vi "TCP Send Recieve.vi"(6 "bytes to read":i32=-1, 7 "mode (standard)":T1(ring), 8 "Error In":errorcluster, 9 "timeout ms (25000)":i32=25000, 10 "data in":string, 11 "connection ID":refnum<k5>) -> (0 "Error Out":errorcluster, 1 "bytes written":i32, 2 "data out":string, 3 "connection ID out":refnum<k5>)   [LabVIEW 2024]
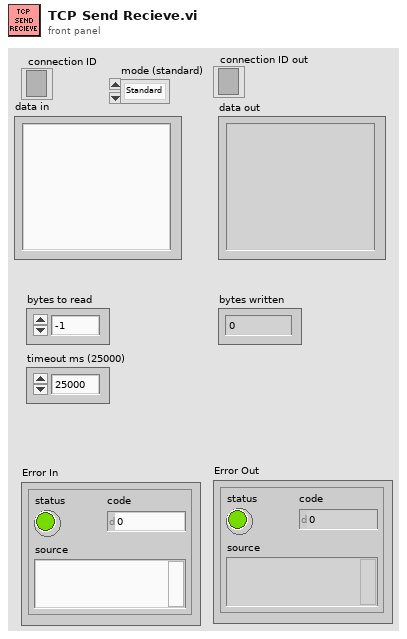
[diagram p1: front panel]
types:
  T1 = enum16{"Standard", "Buffered", "CRLF", "Immediate"}
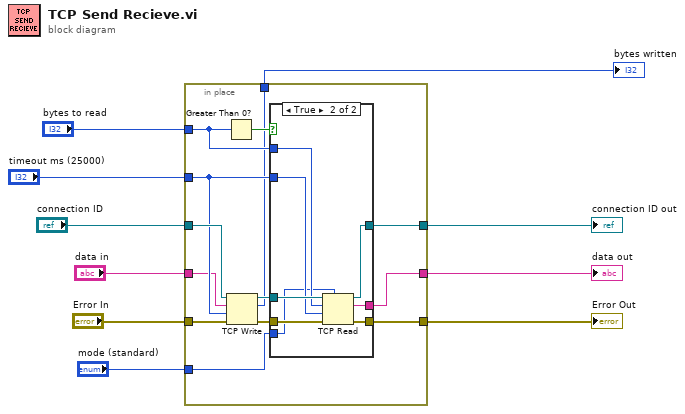
[diagram p0: block diagram]
diagram:
  n1 = in-place {
    in-place-border: [w23] -> w10
    in-place-border: [w22] -> w9
    in-place-border: [w21] -> w8
    in-place-border: "connection ID" -> [w20]
    in-place-border: "Error In" -> [w17]
    in-place-border: "timeout ms (25000)" -> [w16]
    in-place-border: "data in" -> [w15]
    in-place-border: "bytes to read" -> [w14]
    in-place-border: "mode (standard)" -> [w12]
    in-place-border: [w11] -> w1
    n2 = Greater Than 0?(x=w14) -> (x > 0?=w13:bool)
    n3 = TCP Write(connection ID=w20, data in=w15, error in (no error)=w17, 9:w16) -> (connection ID out=w19:refnum<k5>, bytes written=w11:i32, error out=w18:errorcluster)
    n4 = case shown="True" w13 {
      tunnel: [w25 w33] -> w23
      tunnel: [w24 w32] -> w22
      tunnel: [_ w31] -> w21
      tunnel: w19 -> [w25 w30]
      tunnel: w18 -> [w24 w29]
      tunnel: w16 -> [_ w28]
      tunnel: w14 -> [_ w27]
      tunnel: w12 -> [_ w26]
      frame False {
      }
      frame True {
        n5 = TCP Read(connection ID=w30, bytes to read=w27, error in (no error)=w29, 7:w26, 9:w28) -> (connection ID out=w33:refnum<k5>, data out=w31:string, error out=w32:errorcluster)
      }
    }
  }
  "Error Out" <- w9
  "connection ID out" <- w10
  "data out" <- w8
  "bytes written" <- w1
